vi "FTW-JSON-ObjectManip-AddPair.vi"(0 "Input JSON Object":string, 1 "Escape Value to String?":bool=TRUE, 5 "Key":string, 7 "Value":string, 9 "Prepend to Pair":string="\n  ", 11 "error in":errorcluster) -> (4 "Output JSON Object":string, 15 "error out":errorcluster)   [LabVIEW 2012]
uses:
  Regex/FTW-Regex.vi
  FTW-JSON-RegexHeader.vi
  Error/FTW-ERR-ThrowError.vi
  FTW-JSON-Escape.vi
panel:
  # "Inputs"
  # "Outputs"
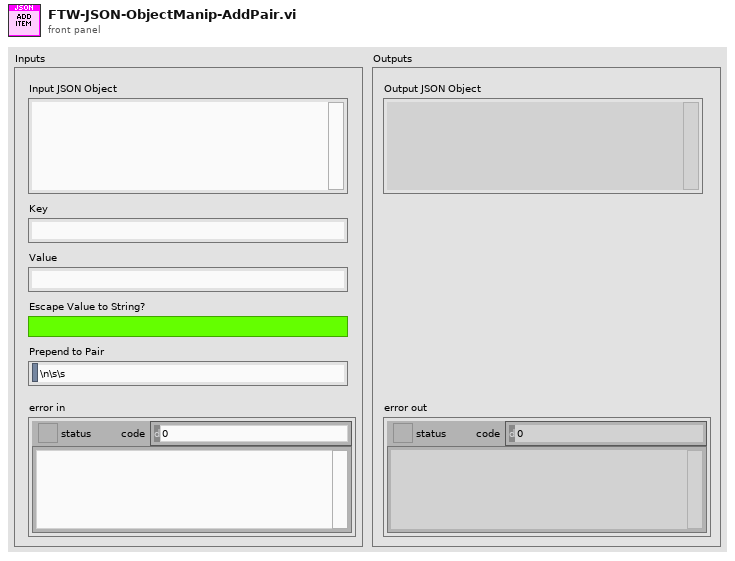
[diagram p1: front panel]
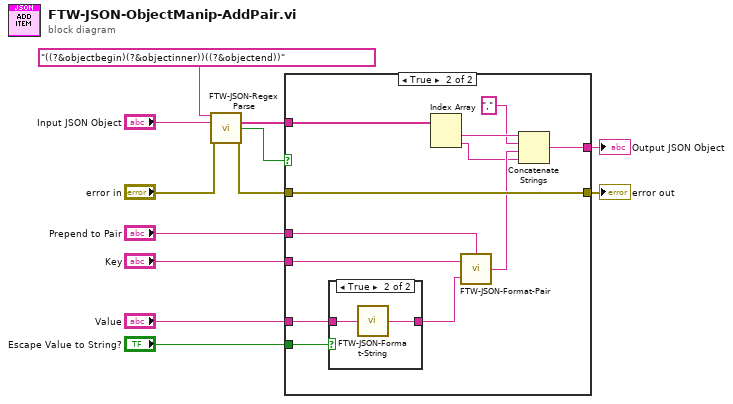
[diagram p0: block diagram]
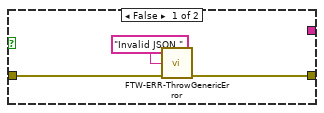
[diagram p2: hidden frame]
diagram:
  n1 = call "FTW-JSON-RegexParse.vi"("Regular Expression using JSON subroutines"="((?&objectbegin)(?&objectinner))((?&objectend))" ("Regular Expression Body"), "Input String"="Input JSON Object", "error in"="error in") -> ("Submatches"=w3:string[], "Found Match?"=w6:bool, "error out"=w4:errorcluster)  [unwired: 8 in, 2 out]
  n2 = case shown="True" w6 {
    tunnel: "Key" -> [_ w27]
    tunnel: "Value" -> [_ w26]
    tunnel: "Escape Value to String?" -> [_ w24]
    tunnel: [w14 w23] -> w5
    tunnel: w4 -> [w15 w23]
    tunnel: w3 -> [_ w22]
    tunnel: [_ w18] -> w2
    tunnel: "Prepend to Pair" -> [_ w17]
    frame False {
      n3 = call "FTW-ERR-ThrowGenericError.vi"("Error Message"="Invalid JSON.", "error in"=w15) -> ("error out"=w14:errorcluster)  [unwired: 13 in]
    }
    frame True {
      n4 = case shown="True" w24 {
        tunnel: w26 -> [w28 w30]
        tunnel: [w28 w29] -> w25
        frame False {
        }
        frame True {
          n5 = call "FTW-JSON-Format-String.vi"("LabVIEW String"=w30) -> ("JSON String"=w29:string)
        }
      }
      n6 = Index Array(array=w22) -> (element #1=w21:string, element #2=w19:string)  [unwired: 2 in]
      n7 = call "FTW-JSON-Format-Pair.vi"("Prepend to Pair"=w17, "Value"=w25, "Key"=w27) -> ("JSON Pair"=w20:string)
      n8 = Concatenate Strings(w21, "," ("string"), w20, w19) -> (w18:string)
    }
  }
  "error out" <- w5
  "Output JSON Object" <- w2
